vi "时间刷新.vi"() -> ()   [LabVIEW 2015]
uses:
  <vilib>/Instr/_visa.llb/VISA Configure Serial Port (Instr).vi
panel:
  in  "VISA资源名称":refnum<visa-resource-name>="COM1"
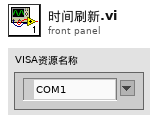
[diagram p1: front panel]
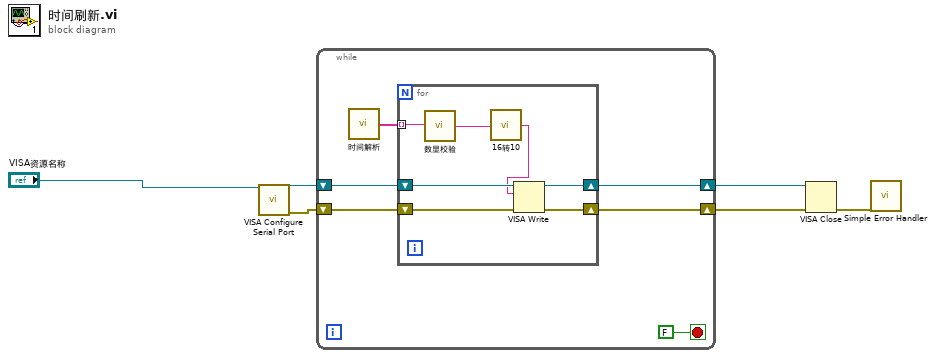
[diagram p0: block diagram]
diagram:
  n1 = call-poly "VISA Configure Serial Port"("VISA resource name"="VISA资源名称") -> ("VISA resource name out"=w4:refnum<visa-resource-name>, "error out"=w5:errorcluster)  [unwired: 8 in, 5 out]
  n2 = while {
    shift-right: [w9] -> w1
    shift-left: w5 -> [w12]
    shift-right: [w10] -> w2
    shift-left: w4 -> [w11]
    stop <- FALSE stop-if-true
    n3 = call "时间解析.vi"() -> ("数组"=w7:string[])
    n4 = for {
      shift-right: [w15] -> w9
      shift-left: w12 -> [w18]
      shift-right: [w16] -> w10
      shift-left: w11 -> [w17]
      tunnel: w7 -> [w13] mode=indexing
      n5 = call "数显校验.vi"("字符串"=w13) -> ("连接的字符串"=w19:string)
      n6 = call "16转10.vi"("字符串"=w19) -> ("字符串 2"=w14:string)
      n7 = VISA Write(VISA resource name=w17, write buffer=w14, error in (no error)=w18) -> (VISA resource name out=w16:refnum<visa-resource-name>, error out=w15:errorcluster)  [unwired: 1 out]
    }
  }
  n8 = VISA Close(VISA resource name=w2, error in (no error)=w1) -> (error out=w3:errorcluster)
  n9 = call <vilib>:"Simple Error Handler.vi"("error in (no error)"=w3) -> ()  [unwired: 1 in, 8 out]
